vi "Close.vi"(8 "error in (no error)":errorcluster, 11 "Avantes in":refnum<class "Avantes.lvclass">) -> (0 "error out":errorcluster, 3 "Avantes out":refnum<class "Avantes.lvclass">)   [LabVIEW 2020, in "Avantes.lvclass"]
uses:
  <instrlib>/Classes/CCD/Avantes/Avantes.lvclass
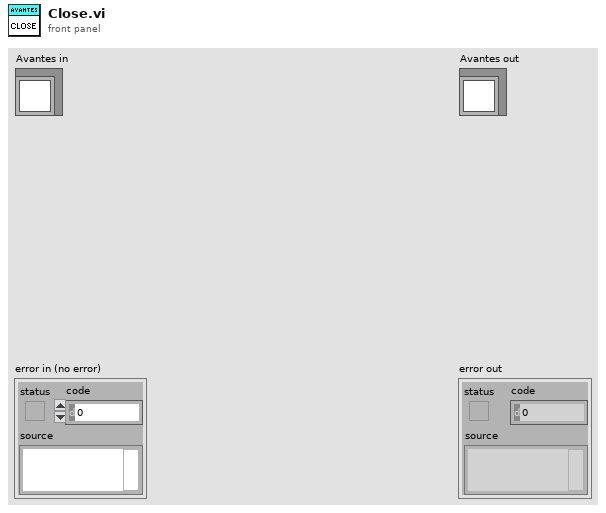
[diagram p1: front panel]
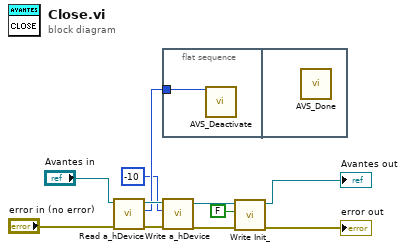
[diagram p0: block diagram]
diagram:
  n1 = call-dynamic "Read a_hDevice.vi"("error in (no error)"="error in (no error)", "Avantes in"="Avantes in") -> ("error out"=w7:errorcluster, "a_hDevice"=w9:i32, "Avantes out"=w11:refnum<class "Avantes.lvclass">)  [unwired: 7 in]
  n2 = flat-sequence {
    tunnel: w9 -> [w12]
    frame #0 {
      n3 = call <instrlib>:"AVS_Deactivate.vi"("a_hHandle"=w12) -> ()  [unwired: 14 in, 1 out]
    }
    frame #1 {
      n4 = call <instrlib>:"AVS_Done.vi"() -> ()  [unwired: 19 in, 1 out]
    }
  }
  n5 = call-dynamic "Write a_hDevice.vi"("error in (no error)"=w7, "a_hDevice"=-10, "Avantes in"=w11) -> ("error out"=w4:errorcluster, "Avantes out"=w5:refnum<class "Avantes.lvclass">)  [unwired: 7 in]
  n6 = call-dynamic "Write Init_.vi"("error in (no error)"=w4, "Init?"=FALSE, "Avantes in"=w5) -> ("error out"=→"error out":errorcluster, "Avantes out"=→"Avantes out":refnum<class "Avantes.lvclass">)  [unwired: 7 in]
